vi "Read channels.vi"(8 "error in (no error)":errorcluster, 11 "Counter Config in":refnum<class "Counter Config.lvclass">) -> (0 "error out":errorcluster, 2 "Channels":refnum<class "TBM channel.lvclass">[](array[class]), 3 "Counter Config out":refnum<class "Counter Config.lvclass">)   [LabVIEW 2015, in "Counter Config.lvclass"]
uses:
  Counter Config.lvclass
  <vilib>/NI/Tag Bus Module Framework/channel/TBM channel.lvclass
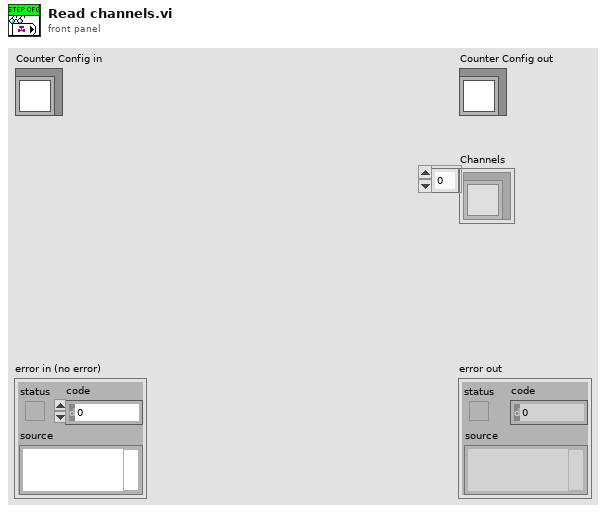
[diagram p1: front panel]
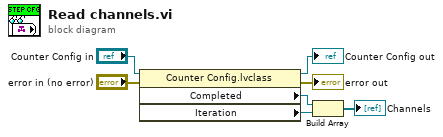
[diagram p0: block diagram]
diagram:
  n1 = property class="Counter Config.lvclass"(reference="Counter Config in", error in="error in (no error)") -> (reference out=→"Counter Config out":refnum<class "Counter Config.lvclass">, error out=→"error out":errorcluster, "Completed"=w3:refnum<class "TBM channel.lvclass">, "Iteration"=w2:refnum<class "TBM channel.lvclass">)
  n2 = Build Array(w3, w2) -> (→"Channels":refnum<class "TBM channel.lvclass">[])
